vi "Step Delete All.vi"(8 "error in (no error)":errorcluster, 10 "sxSequenceId (\"\")":string, 11 "Connection Refnum":T1) -> (0 "error out":errorcluster, 3 "Connection Refnum":T1)   [LabVIEW 2011]
uses:
  Summitek EXT/ODBC/SQL Controls/Connection Refnum.ctl
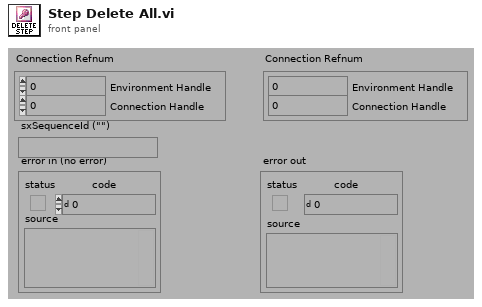
[diagram p1: front panel]
types:
  T1 = typedef "Connection Refnum.ctl" = cluster{"Environment Handle":i32, "Connection Handle":i32}
  T2 = typedef "Step Record.ctl" = cluster{"ixStep":i32, "sxSequenceId":string, "sxTestId":string, "iIndex":i32, "iRepeat":i32, "iQuickMode":i32, "sTag":string, "sDatasheetsCSV":string, "bConfiguration":string}
  T3 = typedef "Statement Refnum.ctl" = cluster{"Statement Handle":i32, "Parameter Number":u16}
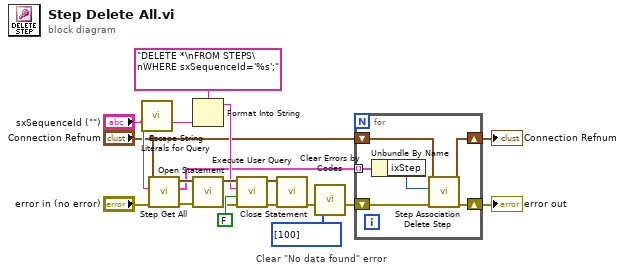
[diagram p0: block diagram]
diagram:
  # "Clear \"No data found\" error"
  n1 = call "Escape String Literals for Query.vi"("String"="sxSequenceId (\"\")") -> ("escaped String"=w10:string)  [unwired: 1 in, 13 out]
  n2 = call "Step Get All.vi"("error in (no error)"="error in (no error)", "sxSequenceId"="sxSequenceId (\"\")", "Connection Refnum"="Connection Refnum") -> ("error out"=w8:errorcluster, "Sequence Steps"=w3:T2[], "Connection Refnum"=w7:T1)  [unwired: 4 in, 2 out]
  n3 = Format Into String(format string="DELETE *\nFROM STEPS\nWHERE sxSequenceId='%s';" ("User Query"), w10) -> (resulting string=w13:string)  [unwired: 2 in, 1 out]
  n4 = call "Open Statement.vi"("error in (no error)"=w8, "Connection Refnum"=w7) -> ("error out"=w15:errorcluster, "Statement Refnum"=w14:T3)  [unwired: 4 out]
  n5 = call "Execute User Query.vi"("error in (no error)"=w15, "Return Data? (f)"=FALSE, "User Query"=w13, "Statement Refnum"=w14) -> ("error out"=w17:errorcluster, "Statement Refnum"=w18:T3)  [unwired: 2 out]
  n6 = call "Close Statement.vi"("error in (no error)"=w17, "Statement Refnum"=w18) -> ("error out"=w12:errorcluster)  [unwired: 5 out]
  n7 = call "Clear Errors by Codes.vi"("Error Codes\nto Clear (Empty)"=i32[] [100] ("Error Codes\nto Clear (Empty)"), "error in (no error)"=w12) -> ("error out"=w5:errorcluster)  [unwired: 5 out]
  n8 = for {
    shift-right: [w20] -> w2
    shift-left: w5 -> [w24]
    shift-right: [w21] -> w1
    shift-left: "Connection Refnum" -> [w25]
    tunnel: w3 -> [w23] mode=indexing
    n9 = Unbundle By Name(w23) -> ("ixStep"=w22:i32)
    n10 = call "Step Association Delete Step.vi"("error in (no error)"=w24, "iStep (0)"=w22, "Connection Refnum"=w25) -> ("error out"=w20:errorcluster, "Connection Refnum"=w21:T1)  [unwired: 7 in]
  }
  "error out" <- w2
  "Connection Refnum" <- w1
